vi "4Pi AA Get Start Position.vi"(0 "Number of Steps":u16, 7 "Center Value":dbl=7.0, 11 "Step Size":dbl) -> (4 "Starting Value":dbl, 15 "Step Size (Dup)":dbl)   [LabVIEW 2020]
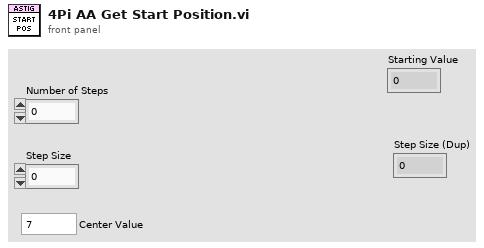
[diagram p1: front panel]
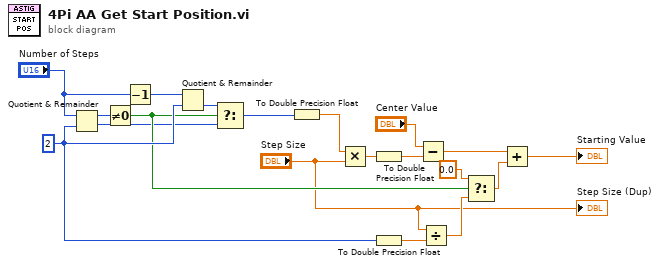
[diagram p0: block diagram]
diagram:
  w18 = u16 2 ("y")
  n1 = Quotient & Remainder(x="Number of Steps", y=w18) -> (x-y*floor(x/y)=w5:u16, floor(x/y)=w8:u16)
  n2 = Not Equal To 0?(x=w5) -> (x != 0?=w17:bool)
  n3 = Decrement(x="Number of Steps") -> (x-1=w6:u16)
  n4 = Quotient & Remainder(x=w6, y=w18) -> (floor(x/y)=w7:u16)  [unwired: 1 out]
  n5 = Select(t=w7, s=w17, f=w8) -> (s? t:f=w9:u16)
  n6 = To Double Precision Float(number=w9) -> (double precision float=w4:dbl)
  n7 = Multiply(x=w4, y="Step Size") -> (x*y=w11:dbl)
  n8 = To Double Precision Float(number=w11) -> (double precision float=w12:dbl)
  n9 = To Double Precision Float(number=w18) -> (double precision float=w19:dbl)
  n10 = Subtract(x="Center Value", y=w12) -> (x-y=w13:dbl)
  n11 = Divide(x="Step Size", y=w19) -> (x/y=w14:dbl)
  n12 = Select(t=0.0, s=w17, f=w14) -> (s? t:f=w15:dbl)
  n13 = Add(x=w13, y=w15) -> (x+y=→"Starting Value":dbl)
  "Step Size (Dup)" <- "Step Size"
